vi "Initialize Image Buffer.vi"(8 "error in (no error)":errorcluster, 11 "Picam in":refnum<class "Picam.lvclass">) -> (0 "error out":errorcluster, 3 "Picam out":refnum<class "Picam.lvclass">)   [LabVIEW 2019, in "Picam.lvclass"]
uses:
  Picam.lvclass
  Picam.lvclass/Picam.ctl
  picam32_LabView_SDK/PICam_lib/PICam.lvlib
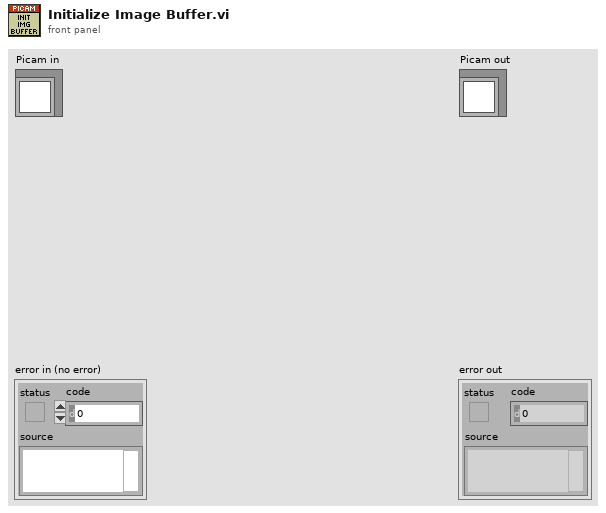
[diagram p1: front panel]
types:
  T1 = typedef "PICam.lvlib/DataAcquisitionResult.ctl" = cluster{"Bytes":u8[], "ReadoutCount":i64, "FramesPerReadout":i32, "Rois":T2[], "PixelBitDepth":i32, "TimeStampBitDepth":i32, "FrameTrackingBitDepth":i32, "GateTrackingBitDepth":i32, "ModulationTrackingBitDepth":i32, "DataHandle":u64}
  T2 = typedef "PicamRoi.ctl" = cluster{"x":i32, "width":i32, "x_binning":i32, "y":i32, "height":i32, "y_binning":i32}
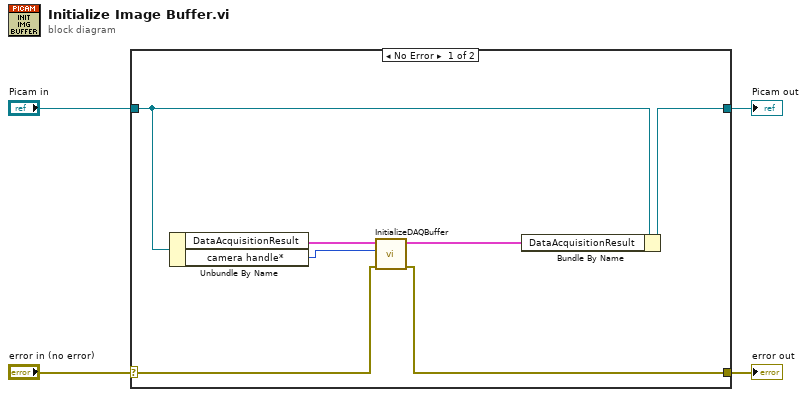
[diagram p0: block diagram]
diagram:
  n1 = case shown="No Error" "error in (no error)" {
    selector: "error in (no error)" -> [w9 w13]
    tunnel: [w8 w13] -> w3
    tunnel: [w6 w12] -> w1
    tunnel: "Picam in" -> [w11 w12]
    frame No Error {
      n2 = Unbundle By Name(w11) -> ("DataAcquisitionResult"=w10:T1, "camera handle*"=w7:u64)
      n3 = call "InitializeDAQBuffer.vi"("error in (no error)"=w9, "PicamHandle (camera)"=w7, "DataAcquisitionBuffer in"=w10) -> ("error out"=w8:errorcluster, "DataAcquisitionBuffer out"=w5:T1)  [unwired: 6 in, 1 out]
      n4 = Bundle By Name(cluster=w11, "DataAcquisitionResult"=w5) -> (w6:refnum<class "Picam.lvclass">)
    }
    frame Error {
    }
  }
  "error out" <- w3
  "Picam out" <- w1
